vi "Get Temperature.vi"(6 "Channel":i32, 8 "error in (no error)":errorcluster, 11 "instrument.Cryostation in":refnum<class "instrument.Cryostation.lvclass">) -> (0 "error out":errorcluster, 1 "Status":variant, 2 "Temperature (K)":dbl, 3 "instrument.Cryostation out":refnum<class "instrument.Cryostation.lvclass">, 4 "Finished?":bool)   [LabVIEW 2016, in "instrument.Cryostation.lvclass"]
uses:
  instrument.Cryostation.lvclass
  Typedefs/Commands-enum.ctl
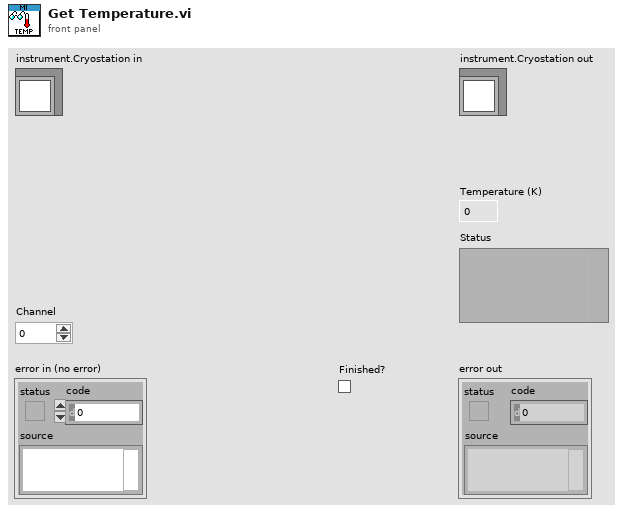
[diagram p1: front panel]
types:
  T1 = typedef "instrument.Cryostation.lvclass/Commands-enum.ctl" = enum16{"Get Temperature", "getAll"}
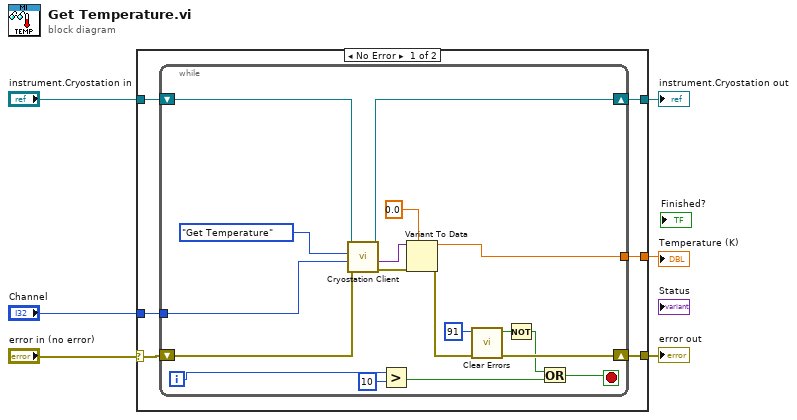
[diagram p0: block diagram]
diagram:
  n1 = case shown="No Error" "error in (no error)" {
    selector: "error in (no error)" -> [w9 w32]
    tunnel: [w12 _] -> w6
    tunnel: [w8 w32] -> w5
    tunnel: [w11 w31] -> w4
    tunnel: "instrument.Cryostation in" -> [w10 w31]
    tunnel: "Channel" -> [w7 _]
    frame No Error {
      n2 = while {
        tunnel: [w14] -> w12
        shift-right: [w29] -> w11
        shift-left: w10 -> [w28]
        shift-right: [w24] -> w8
        shift-left: w9 -> [w25]
        tunnel: w7 -> [w13]
        i -> [w19]
        stop <- w18 stop-if-true
        n3 = call "Cryostation Client.vi"("error in (no error)"=w25, "Data"=w13, "Command"=Commands-enum."Get Temperature", "instrument.Cryostation in"=w28) -> ("error out"=w27:errorcluster, "Data out"=w26:variant, "instrument.Cryostation out"=w29:refnum<class "instrument.Cryostation.lvclass">)  [unwired: 4 in, 1 out]
        n4 = Greater?(x=w19, y=10) -> (0:w20:bool)
        n5 = Variant To Data(error in=w27, type=0.0 ("Temperature (K)"), Variant=w26) -> (data=w14:dbl, error out=w30:errorcluster)
        n6 = call <vilib>:"Clear Errors.vi"("error in (no error)"=w30, "specific error code to clear (0: all)"=91) -> ("error out"=w24:errorcluster, "specific error cleared?"=w17:bool)  [unwired: 4 in]
        n7 = Not(x=w17) -> (.not. x?=w16:bool)
        n8 = Or(x=w16, y=w20) -> (x .or. y?=w18:bool)
      }
    }
    frame Error {
    }
  }
  "error out" <- w5
  "instrument.Cryostation out" <- w4
  "Temperature (K)" <- w6
